vi "Send Signal.vi"(8 "error in":errorcluster, 10 "Input":variant, 11 "PCAN in":refnum<class "PCAN.lvclass">) -> (0 "error out":errorcluster, 3 "PCAN out":refnum<class "PCAN.lvclass">)   [LabVIEW 2023, in "PCAN.lvclass"]
uses:
  PCAN.lvclass
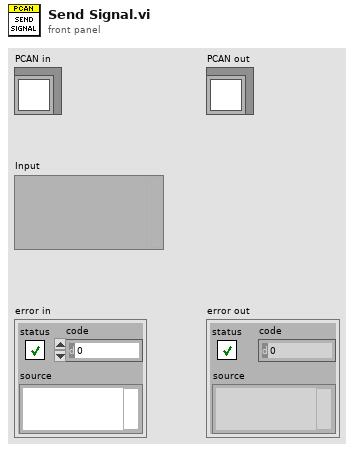
[diagram p1: front panel]
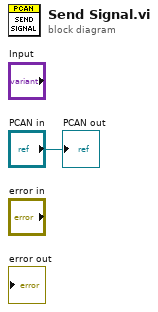
[diagram p0: block diagram]
diagram:
  "PCAN out" <- "PCAN in"
